vi "niRFUtil WFM Quad Fit Fine Align (complex wfm).vi"(0 "Acquired Waveform In":T1={"x0"=0.0, "dx"=1.0, "y"=[]} {"y" format="%.2f"; "dx" format="%^.2e"; "x0" format="%^.2e"}, 1 "Reference Waveform In":T1={"x0"=0.0, "dx"=1.0, "y"=[]} {"y" format="%.2f"; "dx" format="%^.2e"; "x0" format="%^.2e"}, 2 "Window Start (s)":dbl=-inf format="%.2p", 3 "Window Duration (s)":dbl=1e-05 format="%.2p", 4 "Half Length":i32=5 format="%.0g", 5 "error in":errorcluster) -> (14 "Acqured Waveform Out":T1 {"y" format="%.2f"; "dx" format="%^.2e"; "x0" format="%^.2e"}, 15 "Reference Waveform Out":T1 {"y" format="%.2f"; "dx" format="%^.2e"; "x0" format="%^.2e"}, 19 "error out":errorcluster)   [LabVIEW 2015, in "niRFUtil.lvlib"]
uses:
  niRFUtil.lvlib
  Includes/niRFUtil INC Complex Waveform.ctl
  Includes/niRFUtil INC Complex Array.ctl
  <vilib>/Analysis/6fits.llb/Curve Fitting Criteria.ctl
  niRFUtil WFM Complex Differential (complex wfm).vi
  niRFUtil WFM Parse Waveform - Duration (complex wfm).vi
  <vilib>/Analysis/NI_AALPro.lvlib
  Includes/niRFUtil INC Real Array.ctl
  Includes/niRFUtil INC Real Waveform.ctl
  <vilib>/Analysis/5stat.llb/RMS (DBL).vi
  niRFUtil WFM Parse Waveform - Duration (real wfm).vi
panel:
  out "Aligned EVM(dB)":dbl
  out "Unaligned EVM(dB)":dbl
  out "Unaligned":cluster{"x0":dbl, "dx":dbl, "y":sgl[]}[](graph)
  out "Aligned":cluster{"x0":dbl, "dx":dbl, "y":sgl[]}[](graph)
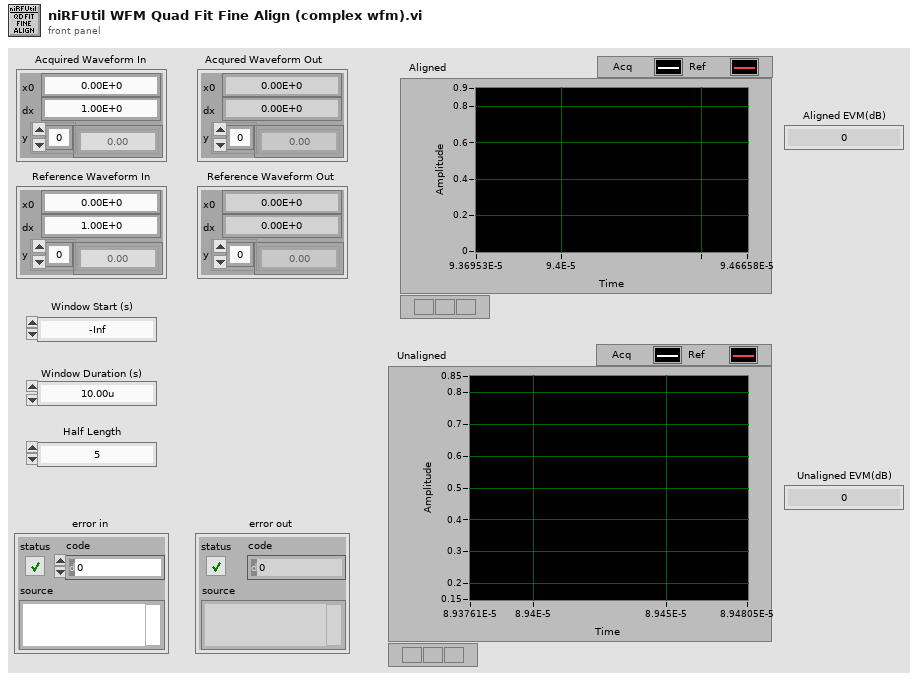
[diagram p1: front panel]
types:
  T1 = typedef "niRFUtil.lvlib/niRFUtil INC Complex Waveform.ctl" = cluster{"x0":dbl, "dx":dbl, "y":T2}
  T2 = typedef "niRFUtil.lvlib/niRFUtil INC Complex Array.ctl" = csg[]
  T3 = typedef "NI_AALPro.lvlib/Curve Fitting Criteria.ctl" = u16
  T4 = typedef "niRFUtil.lvlib/niRFUtil INC Real Waveform.ctl" = cluster{"x0":dbl, "dx":dbl, "y":T5}
  T5 = typedef "niRFUtil.lvlib/niRFUtil INC Real Array.ctl" = sgl[]
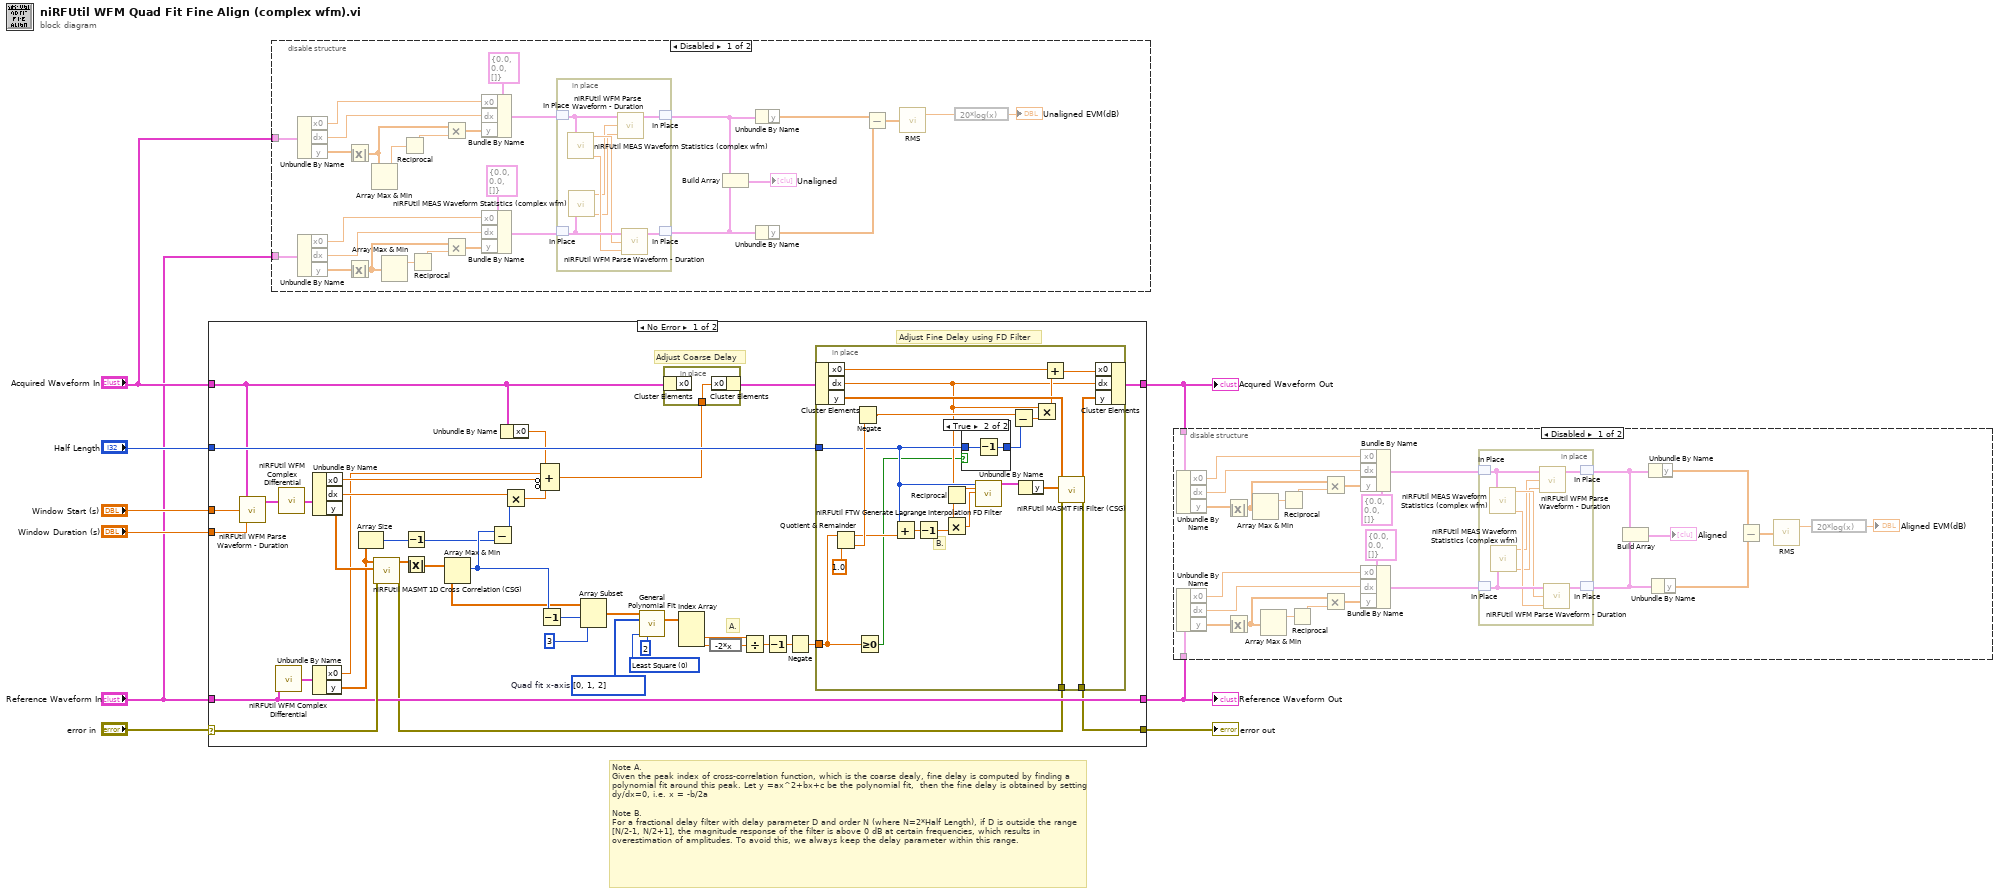
[diagram p0: block diagram]
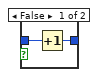
[diagram p4: hidden frame]
diagram:
  # "Note A.\nGiven the peak index of cross-correlation function, which is the coarse dealy, fine delay is computed by finding a polynomial fit around this peak. Let y =ax^2+bx+c be the polynomial fit,  then the fine delay is obtained by setting dy/dx=0, i.e. x = -b/2a\n\nNote B.\nFor a fractional delay filter with delay parameter D and order N (where N=2*Half Length), if D is outside the range [N/2-1, N/2+1], the magnitude response of the filter is above 0 dB at certain frequencies, which results in overestimation of amplitudes. To avoid this, we always keep the delay parameter within this range."
  n1 = case shown="No Error" "error in" {
    selector: "error in" -> [w38 w80]
    tunnel: "Window Duration (s)" -> [w34 _]
    tunnel: "Reference Waveform In" -> [w30 w78]
    tunnel: [w30 w78] -> w3
    tunnel: "Acquired Waveform In" -> [w22 w79]
    tunnel: [w27 w79] -> w4
    tunnel: "Half Length" -> [w40 _]
    tunnel: [w28 w80] -> w6
    tunnel: "Window Start (s)" -> [w37 _]
    frame No Error {
      w26 = i32[] [0, 1, 2]  # Quad fit x-axis
      w42 = T3 0 items=["Least Square", "Least Absolute Residual", "Bisquare"] ("method")
      # "Adjust Fine Delay using FD Filter"
      # "Adjust Coarse Delay"
      # "A."
      n2 = call-poly "niRFUtil WFM Parse Waveform - Duration.vi"("Duration (Inf)"=w34, "Start (-Inf)"=w37, "Waveform In"=w22) -> ("Waveform Out"=w36:T1)  [unwired: 2 out]
      n3 = call-poly "niRFUtil WFM Complex Differential.vi"("Waveform In"=w30) -> ("Waveform Out"=w33:T1)  [unwired: 14 out]
      n4 = call-poly "niRFUtil WFM Complex Differential.vi"("Waveform In"=w36) -> ("Waveform Out"=w35:T1)  [unwired: 14 out]
      n5 = Unbundle By Name(w35) -> ("x0"=w12:dbl, "dx"=w14:dbl, "y"=w32:T2)
      n6 = Unbundle By Name(w33) -> ("x0"=w10:dbl, "y"=w11:T2)
      n7 = Array Size(array=w11) -> (size(s)=w16:i32)
      n8 = call "niRFUtil MASMT 1D Cross Correlation (CSG).vi"("error in (no error)"=w38, "Y"=w32, "X"=w11) -> ("error out"=w29:errorcluster, "Rxy"=w39:csg[])  [unwired: 7 in]
      n9 = Decrement(x=w16) -> (x-1=w15:i32)
      n10 = Absolute Value(x=w39) -> (abs(x)=w17:sgl[])
      n11 = Array Max & Min(array=w17) -> (max index (indices)=w24:i32)  [unwired: 3 out]
      n12 = Subtract(x=w24, y=w15) -> (x-y=w23:i32)
      n13 = Unbundle By Name(w22) -> ("x0"=w21:dbl)
      n14 = Multiply(x=w14, y=w23) -> (x*y=w13:dbl)
      n15 = Decrement(x=w24) -> (x-1=w47:i32)
      n16 = Compound Arithmetic op=ADD(w21, w10, invert w12, invert w13) -> (w20:dbl)
      n17 = Array Subset(array=w17, index=w47, length=3) -> (w49:sgl[])
      n18 = call <vilib>:"General Polynomial Fit.vi"("Y"=w49, "polynomial order"=2, "X"=w26, "method"=w42) -> ("Polynomial Coefficients"=w43:dbl[])  [unwired: 8 in, 3 out]
      n19 = in-place {
        in-place-border: w20 -> [w50]
        n20 = in-place-cluster #1(w22) -> ()  [unwired: 1 out]
        n21 = in-place-cluster #1("x0"=w50) -> (w25:T1)
      }
      n22 = Index Array(array=w43) -> (element #2=w44:dbl, element #3=w45:dbl)  [unwired: 3 in, 1 out]
      n23 = expression code="-2*x"(w45) -> (w46:dbl)
      n24 = Divide(x=w44, y=w46) -> (x/y=w48:dbl)
      n25 = Decrement(x=w48) -> (x-1=w19:dbl)
      n26 = Negate(x=w19) -> (-x=w18:dbl)
      n27 = in-place {
        in-place-border: w40 -> [w61]
        in-place-border: w29 -> [w69]
        in-place-border: [w68] -> w28
        in-place-border: w18 -> [w62]
        # "B."
        n28 = in-place-cluster #2(w25) -> ("x0"=w64:dbl, "dx"=w59:dbl, "y"=w67:T2)
        n29 = Quotient & Remainder(x=w62, y=1.0) -> (x-y*floor(x/y)=w54:dbl, floor(x/y)=w63:dbl)
        n30 = Negate(x=w63) -> (-x=w60:dbl)
        n31 = Greater Or Equal To 0?(x=w62) -> (x >= 0?=w53:bool)
        n32 = Add(x=w61, y=w54) -> (x+y=w71:dbl)
        n33 = Decrement(x=w71) -> (x-1=w70:dbl)
        n34 = Reciprocal(x=w59) -> (1/x=w52:dbl)
        n35 = Multiply(x=w59, y=w70) -> (x*y=w51:dbl)
        n36 = case shown="True" w53 {
          tunnel: w61 -> [w75 w77]
          tunnel: [w74 w76] -> w55
          frame False {
            n37 = Increment(x=w75) -> (x+1=w74:i32)
          }
          frame True {
            n38 = Decrement(x=w77) -> (x-1=w76:i32)
          }
        }
        n39 = call "niRFUtil FTW Generate Lagrange Interpolation FD Filter.vi"("Half Length"=w61, "Sampling Rate (Hz)"=w52, "Delay (s)"=w51) -> ("Filter"=w73:T4)  [unwired: 16 in]
        n40 = Subtract(x=w60, y=w55) -> (x-y=w56:dbl)
        n41 = Unbundle By Name(w73) -> ("y"=w72:T5)
        n42 = Multiply(x=w59, y=w56) -> (x*y=w65:dbl)
        n43 = Add(x=w64, y=w65) -> (x+y=w58:dbl)
        n44 = call "niRFUtil MASMT FIR Filter (CSG).vi"("error in (no error)"=w69, "FIR Coefficients"=w72, "X"=w67) -> ("error out"=w68:errorcluster, "Filtered X"=w57:csg[])  [unwired: 7 in]
        n45 = in-place-cluster #2("x0"=w58, "dx"=w59, "y"=w57) -> (w27:T1)
      }
    }
    frame Error {
    }
  }
  "Reference Waveform Out" <- w3
  "Acqured Waveform Out" <- w4
  "error out" <- w6
  n46 = disable-structure shown="Disabled" {
    disable-tunnel: "Acquired Waveform In" -> [w93 _]
    disable-tunnel: "Reference Waveform In" -> [w92 _]
    frame Disabled {
      n47 = Unbundle By Name(w93) -> ("x0"=w106:dbl, "dx"=w105:dbl, "y"=w95:T2)
      n48 = Unbundle By Name(w92) -> ("x0"=w107:dbl, "dx"=w108:dbl, "y"=w103:T2)
      n49 = Absolute Value(x=w95) -> (abs(x)=w97:sgl[])
      n50 = Absolute Value(x=w103) -> (abs(x)=w101:sgl[])
      n51 = Array Max & Min(array=w97) -> (max value=w96:sgl)  [unwired: 3 out]
      n52 = Array Max & Min(array=w101) -> (max value=w102:sgl)  [unwired: 3 out]
      n53 = Reciprocal(x=w96) -> (1/x=w98:sgl)
      n54 = Reciprocal(x=w102) -> (1/x=w100:sgl)
      n55 = Multiply(x=w97, y=w98) -> (x*y=w91:sgl[])
      n56 = Multiply(x=w101, y=w100) -> (x*y=w90:sgl[])
      n57 = Bundle By Name(cluster=T4 {"x0"=0.0, "dx"=0.0, "y"=[]} ("input cluster"), "x0"=w106, "dx"=w105, "y"=w91) -> (w85:T4)
      n58 = Bundle By Name(cluster=T4 {"x0"=0.0, "dx"=0.0, "y"=[]} ("input cluster"), "x0"=w107, "dx"=w108, "y"=w90) -> (w86:T4)
      n59 = in-place {
        n60 = in-place-match #3(w85) -> (w114:T4)
        n61 = in-place-match #4(w86) -> (w113:T4)
        n62 = call "niRFUtil MEAS Waveform Statistics (complex wfm).vi"("Waveform In"=w114) -> ("Start"=w112:dbl, "Duration"=w111:dbl)  [unwired: 4 in, 2 out]
        n63 = call "niRFUtil MEAS Waveform Statistics (complex wfm).vi"("Waveform In"=w113) -> ("Start"=w110:dbl, "Duration"=w109:dbl)  [unwired: 4 in, 2 out]
        n64 = call-poly "niRFUtil WFM Parse Waveform - Duration.vi"("Duration (Inf)"=w109, "Start (-Inf)"=w110, "Waveform In"=w114) -> ("Waveform Out"=w115:T4)  [unwired: 2 in]
        n65 = call-poly "niRFUtil WFM Parse Waveform - Duration.vi"("Duration (Inf)"=w111, "Start (-Inf)"=w112, "Waveform In"=w113) -> ("Waveform Out"=w116:T4)  [unwired: 2 in]
        n66 = in-place-match #3(w115) -> (w84:T4)
        n67 = in-place-match #4(w116) -> (w82:T4)
      }
      n68 = Build Array(w84, w82) -> (→"Unaligned":T4[])
      n69 = Unbundle By Name(w84) -> ("y"=w83:T5)
      n70 = Unbundle By Name(w82) -> ("y"=w81:T5)
      n71 = Subtract(x=w83, y=w81) -> (x-y=w89:T5)
      n72 = call-poly <vilib>:"RMS.vi"("X"=w89) -> ("rms value"=w88:dbl)  [unwired: 1 out]
      n73 = expression code="20*log(x)"(w88) -> (→"Unaligned EVM(dB)":dbl)
    }
    frame Enabled {
    }
  }
  n74 = disable-structure shown="Disabled" {
    disable-tunnel: w4 -> [w143 _]
    disable-tunnel: w3 -> [w134 _]
    frame Disabled {
      n75 = Unbundle By Name(w143) -> ("x0"=w130:dbl, "dx"=w131:dbl, "y"=w142:T2)
      n76 = Unbundle By Name(w134) -> ("x0"=w129:dbl, "dx"=w128:dbl, "y"=w133:T2)
      n77 = Absolute Value(x=w142) -> (abs(x)=w140:sgl[])
      n78 = Absolute Value(x=w133) -> (abs(x)=w136:sgl[])
      n79 = Array Max & Min(array=w140) -> (max value=w141:sgl)  [unwired: 3 out]
      n80 = Array Max & Min(array=w136) -> (max value=w135:sgl)  [unwired: 3 out]
      n81 = Reciprocal(x=w141) -> (1/x=w139:sgl)
      n82 = Reciprocal(x=w135) -> (1/x=w137:sgl)
      n83 = Multiply(x=w140, y=w139) -> (x*y=w124:sgl[])
      n84 = Multiply(x=w136, y=w137) -> (x*y=w123:sgl[])
      n85 = Bundle By Name(cluster=T4 {"x0"=0.0, "dx"=0.0, "y"=[]} ("input cluster"), "x0"=w130, "dx"=w131, "y"=w124) -> (w122:T4)
      n86 = Bundle By Name(cluster=T4 {"x0"=0.0, "dx"=0.0, "y"=[]} ("input cluster"), "x0"=w129, "dx"=w128, "y"=w123) -> (w117:T4)
      n87 = in-place {
        n88 = in-place-match #5(w122) -> (w150:T4)
        n89 = in-place-match #6(w117) -> (w149:T4)
        n90 = call "niRFUtil MEAS Waveform Statistics (complex wfm).vi"("Waveform In"=w150) -> ("Start"=w148:dbl, "Duration"=w147:dbl)  [unwired: 4 in, 2 out]
        n91 = call "niRFUtil MEAS Waveform Statistics (complex wfm).vi"("Waveform In"=w149) -> ("Start"=w146:dbl, "Duration"=w145:dbl)  [unwired: 4 in, 2 out]
        n92 = call-poly "niRFUtil WFM Parse Waveform - Duration.vi"("Duration (Inf)"=w145, "Start (-Inf)"=w146, "Waveform In"=w150) -> ("Waveform Out"=w151:T4)  [unwired: 2 in]
        n93 = call-poly "niRFUtil WFM Parse Waveform - Duration.vi"("Duration (Inf)"=w147, "Start (-Inf)"=w148, "Waveform In"=w149) -> ("Waveform Out"=w152:T4)  [unwired: 2 in]
        n94 = in-place-match #5(w151) -> (w121:T4)
        n95 = in-place-match #6(w152) -> (w120:T4)
      }
      n96 = Build Array(w121, w120) -> (→"Aligned":T4[])
      n97 = Unbundle By Name(w121) -> ("y"=w119:T5)
      n98 = Unbundle By Name(w120) -> ("y"=w118:T5)
      n99 = Subtract(x=w119, y=w118) -> (x-y=w125:T5)
      n100 = call-poly <vilib>:"RMS.vi"("X"=w125) -> ("rms value"=w126:dbl)  [unwired: 1 out]
      n101 = expression code="20*log(x)"(w126) -> (→"Aligned EVM(dB)":dbl)
    }
    frame Enabled {
    }
  }
